vi "Update Limit(User Event).vi"(8 "error in (no error)":errorcluster, 10 "X Range Change User Event Data":T1, 11 "XYGraphOverview in":refnum<class "XYGraphOverview.lvclass">) -> (0 "error out":errorcluster, 3 "XYGraphOverview out":refnum<class "XYGraphOverview.lvclass">)   [LabVIEW 2020, in "XYGraphOverview.lvlib" / "XYGraphOverview.lvclass"]
uses:
  XYGraphOverview.lvclass
  X Range Change User Event Data.ctl
  XYGraphOverview.lvclass/XYGraphOverview.ctl
  Read Block Color.vi
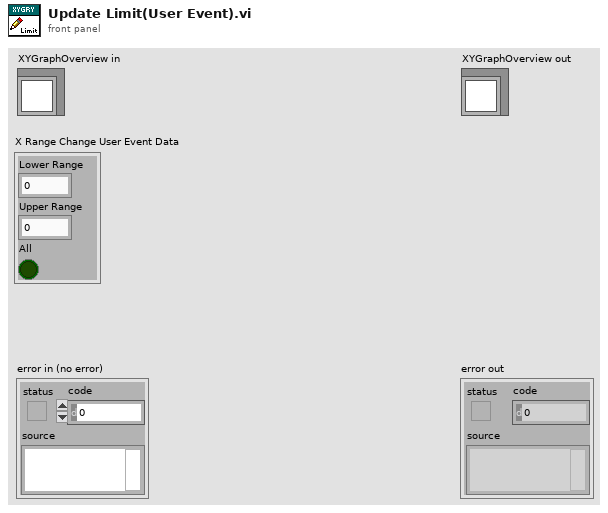
[diagram p1: front panel]
types:
  T1 = typedef "XYGraphOverview.lvlib/XYGraphOverview.lvclass/X Range Change User Event Data.ctl" = cluster{"Lower Range":dbl, "Upper Range":dbl, "All":bool}
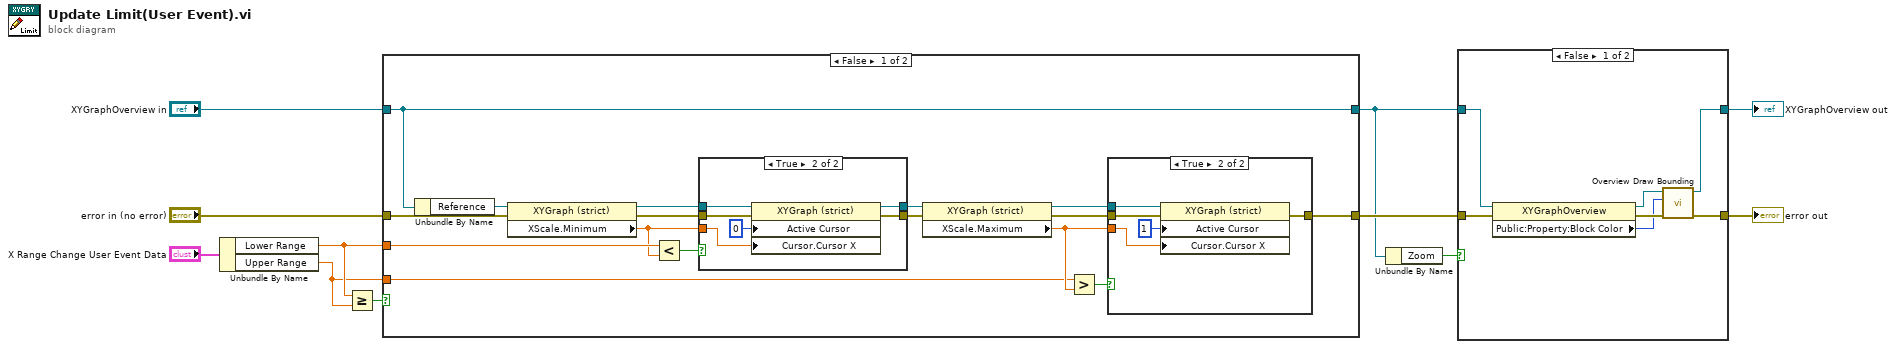
[diagram p0: block diagram]
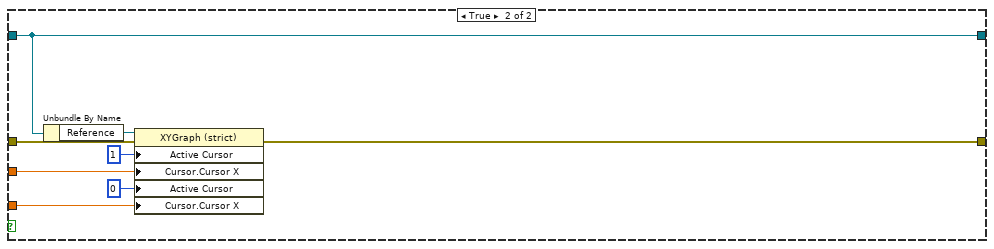
[diagram p5: hidden frame]
diagram:
  n1 = Unbundle By Name("X Range Change User Event Data") -> ("Lower Range"=w7:dbl, "Upper Range"=w6:dbl)
  n2 = Greater Or Equal?(x=w7, y=w6) -> (x >= y?=w11:bool)
  n3 = case shown="False" w11 {
    tunnel: "error in (no error)" -> [w27 w49]
    tunnel: w6 -> [w15 w47]
    tunnel: w7 -> [w26 w44]
    tunnel: [w14 w45] -> w5
    tunnel: "XYGraphOverview in" -> [w13 w43]
    tunnel: [w13 w43] -> w3
    frame False {
      n4 = Unbundle By Name(w13) -> ("Reference"=w12:refnum<vi>)
      n5 = property on="Property Node" class="XYGraph (strict)"(reference=w12, error in=w27) -> (reference out=w23:refnum<vi>, error out=w22:errorcluster, "XScale.Minimum"=w24:dbl)
      n6 = Less?(x=w26, y=w24) -> (x < y?=w25:bool)
      n7 = case shown="True" w25 {
        tunnel: w22 -> [w35 w41]
        tunnel: w23 -> [w34 w40]
        tunnel: w24 -> [_ w38]
        tunnel: [w35 w37] -> w17
        tunnel: [w34 w36] -> w16
        frame False {
        }
        frame True {
          n8 = property class="XYGraph (strict)"(reference=w40, error in=w41, "Active Cursor"=u32 0, "Cursor.Cursor X"=w38) -> (reference out=w36:refnum<vi>, error out=w37:errorcluster)
        }
      }
      n9 = property on="Property Node" class="XYGraph (strict)"(reference=w16, error in=w17) -> (reference out=w20:refnum<vi>, error out=w21:errorcluster, "XScale.Maximum"=w19:dbl)
      n10 = Greater?(x=w15, y=w19) -> (0:w18:bool)
      n11 = case shown="True" w18 {
        tunnel: w21 -> [w28 w33]
        tunnel: w20 -> [_ w32]
        tunnel: w19 -> [_ w30]
        tunnel: [w28 w29] -> w14
        frame False {
        }
        frame True {
          n12 = property class="XYGraph (strict)"(reference=w32, error in=w33, "Active Cursor"=u32 1, "Cursor.Cursor X"=w30) -> (error out=w29:errorcluster)  [unwired: 1 out]
        }
      }
    }
    frame True {
      n13 = Unbundle By Name(w43) -> ("Reference"=w42:refnum<vi>)
      n14 = property class="XYGraph (strict)"(reference=w42, error in=w49, "Active Cursor"=u32 1, "Cursor.Cursor X"=w44, "Active Cursor"=u32 0, "Cursor.Cursor X"=w47) -> (error out=w45:errorcluster)  [unwired: 1 out]
    }
  }
  n15 = Unbundle By Name(w3) -> ("Zoom"=w4:bool)
  n16 = case shown="False" w4 {
    tunnel: w5 -> [w53 w57]
    tunnel: w3 -> [w52 w58]
    tunnel: [w50 w58] -> w2
    tunnel: [w51 w57] -> w1
    frame False {
      n17 = property class="XYGraphOverview"(reference=w52, error in=w53) -> (reference out=w55:refnum<class "XYGraphOverview.lvclass">, error out=w56:errorcluster, "Public:Property:Block Color"=w54:u32)
      n18 = call "Overview Draw Bounding.vi"("error in (no error)"=w56, "Color"=w54, "XYGraphOverview in"=w55) -> ("error out"=w51:errorcluster, "XYGraphOverview out"=w50:refnum<class "XYGraphOverview.lvclass">)  [unwired: 7 in]
    }
    frame True {
    }
  }
  "error out" <- w1
  "XYGraphOverview out" <- w2
